vi "Retrieve Text.vi"(8 "error in (no error)":errorcluster, 11 "xwpfWriter in":refnum<class "xwpfWriter.lvclass">) -> (0 "error out":errorcluster, 2 "Text":string, 3 "xwpfWriter out":refnum<class "xwpfWriter.lvclass">)   [LabVIEW 2017, in "LabVIEW NPOI.lvlib" / "xwpfWriter.lvclass"]
uses:
  xwpfWriter.lvclass
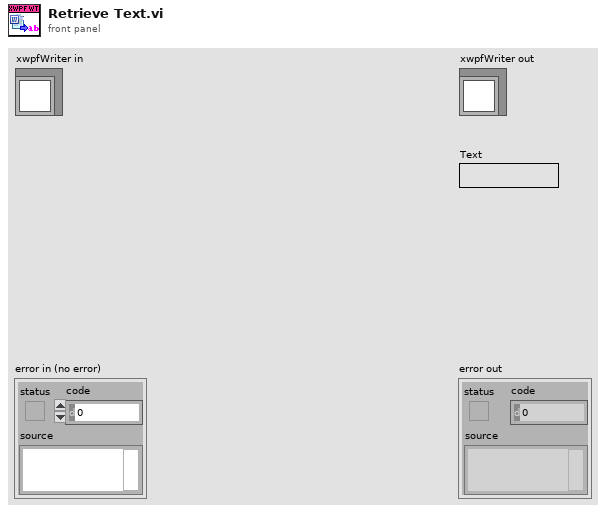
[diagram p1: front panel]
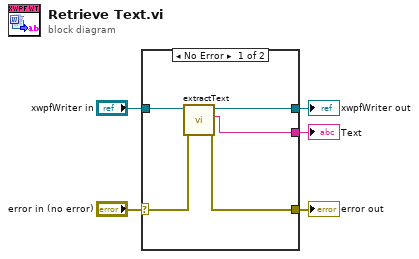
[diagram p0: block diagram]
diagram:
  n1 = case shown="No Error" "error in (no error)" {
    selector: "error in (no error)" -> [w8 w12]
    tunnel: [w7 w12] -> w4
    tunnel: [w9 w11] -> w2
    tunnel: "xwpfWriter in" -> [w10 w11]
    tunnel: [w6 _] -> w1
    frame No Error {
      n2 = call "extractText.vi"("error in (no error)"=w8, "xwpfWriter in"=w10) -> ("error out"=w7:errorcluster, "Text"=w6:string, "xwpfWriter out"=w9:refnum<class "xwpfWriter.lvclass">)  [unwired: 7 in]
    }
    frame Error {
    }
  }
  "error out" <- w4
  "xwpfWriter out" <- w2
  "Text" <- w1
